vi "Configure S-parameter Magnitude-Phase Pairs.vi"(7 "S-parameter Table Name (\"DEFAULT\")":string="DEFAULT", 8 "error in (no error)":errorcluster, 9 "Magnitude Phase Pairs":dbl[](array[numeric]), 10 "S-parameter Type (0: S11)":i32(ring) items=["S11", "S12", "S21", "S22"], 11 "VISA resource name":refnum<visa-resource-name>) -> (0 "error out":errorcluster, 3 "VISA resource name out":refnum<visa-resource-name>)   [LabVIEW 2018, in "Agilent U2000 Series.lvlib"]
doc: "Sets the magnitude-phase pairs for the selected S-parameter type for the\ncurrently selected S-parameter table.\n\nNote:\nThis VI is only applicable for U2040 X-Series."
uses:
  Agilent U2000 Series.lvlib
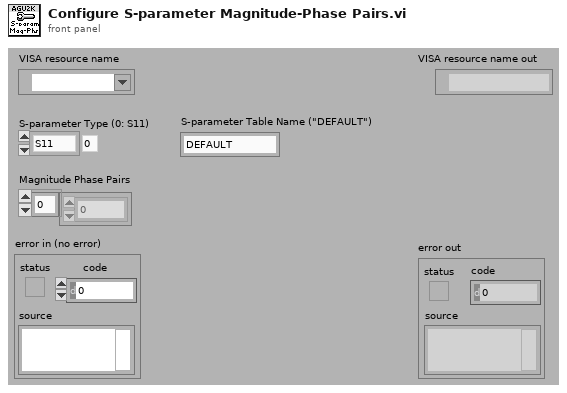
[diagram p1: front panel]
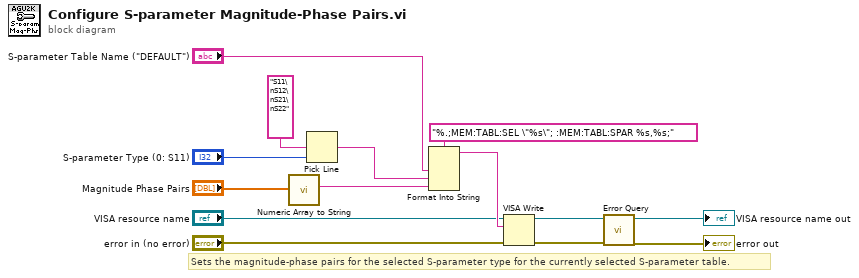
[diagram p0: block diagram]
diagram:
  # "Sets the magnitude-phase pairs for the selected S-parameter type for the currently selected S-parameter table."
  n1 = call "Numeric Array to String.vi"("List Data"="Magnitude Phase Pairs") -> ("Result String"=w1:string)  [unwired: 10 out]
  n2 = Pick Line(multi-line string="S11\nS12\nS21\nS22", line index="S-parameter Type (0: S11)") -> (output string=w2:string)  [unwired: 1 in]
  n3 = Format Into String(format string="%.;MEM:TABL:SEL \"%s\"; :MEM:TABL:SPAR %s,%s;", "S-parameter Table Name (\"DEFAULT\")", w2, w1) -> (resulting string=w13:string)  [unwired: 2 in, 1 out]
  n4 = VISA Write(VISA resource name="VISA resource name", write buffer=w13, error in (no error)="error in (no error)") -> (VISA resource name out=w10:refnum<visa-resource-name>, error out=w9:errorcluster)  [unwired: 1 out]
  n5 = call "Error Query.vi"("error in (no error)"=w9, "VISA resource name"=w10) -> ("error out"=→"error out":errorcluster, "VISA resource name out"=→"VISA resource name out":refnum<visa-resource-name>)  [unwired: 6 in, 2 out]
